vi "Generate Gene.vi"(8 "error in":errorcluster, 11 "Bit in":refnum<class "Bit.lvclass">) -> (0 "error out":errorcluster, 3 "Bit out":refnum<class "Bit.lvclass">)   [LabVIEW 2016, in "Bit.lvclass"]
uses:
  Bit.lvclass
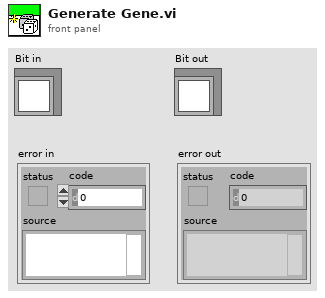
[diagram p1: front panel]
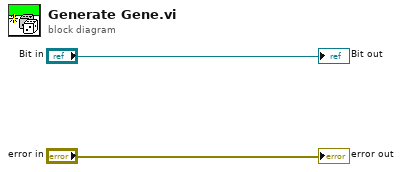
[diagram p0: block diagram]
diagram:
  "error out" <- "error in"
  "Bit out" <- "Bit in"
